vi "Accident Generator.vi"(10 "Accident Number":i32, 11 "Map":i32[][](array[numeric])) -> (2 "Accident Position":T1[](array[typedef]), 3 "Map Out":i32[][](array[numeric]))   [LabVIEW 2015]
uses:
  Data Def/Accident Position.ctl
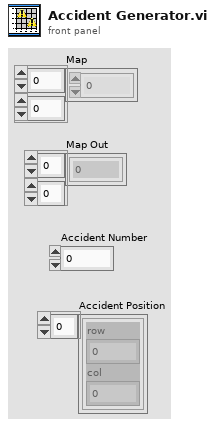
[diagram p1: front panel]
types:
  T1 = typedef "Accident Position.ctl" = cluster{"row":i32, "col":i32}
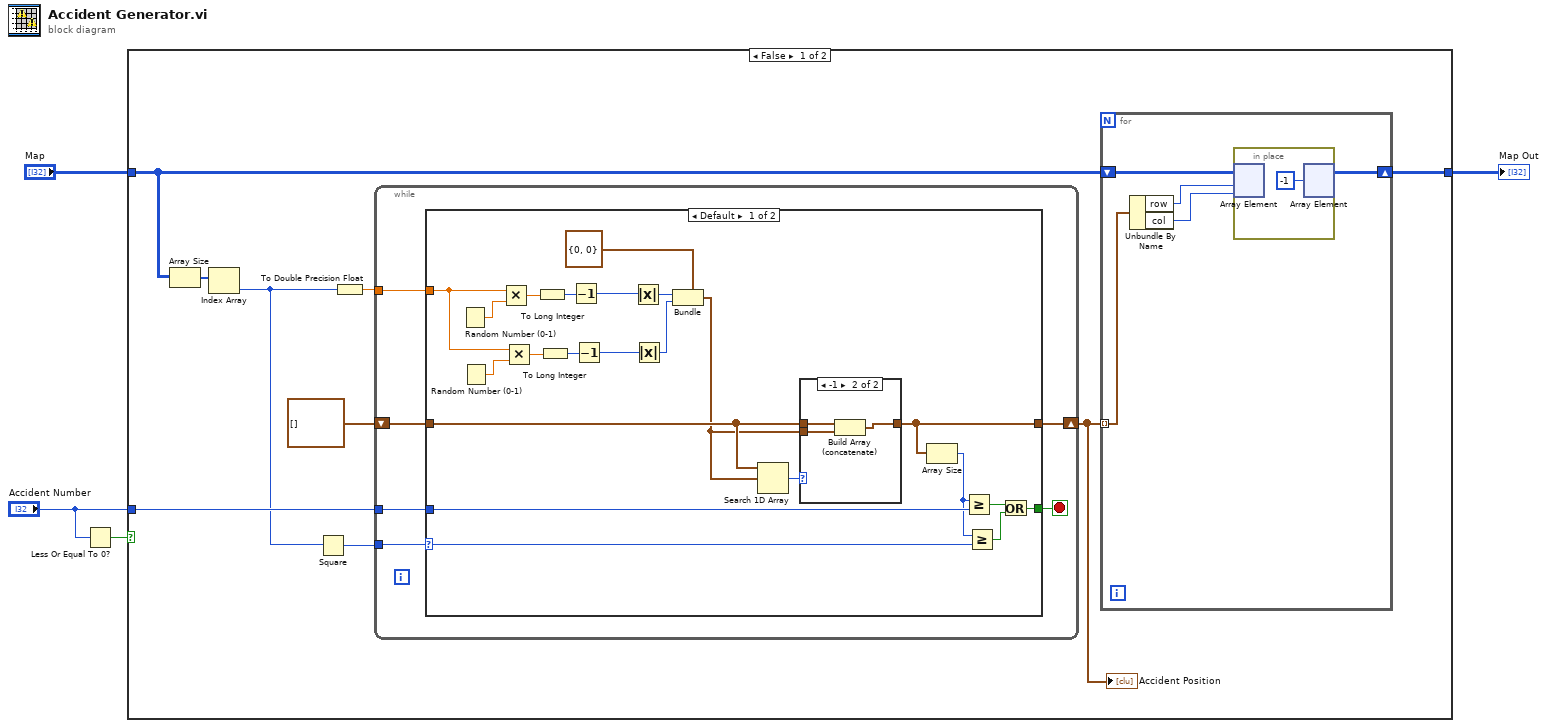
[diagram p0: block diagram]
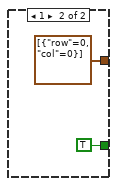
[diagram p3: hidden frame]
diagram:
  n1 = Less Or Equal To 0?(x="Accident Number") -> (x <= 0?=w2:bool)
  n2 = case shown="False" w2 {
    tunnel: "Accident Number" -> [w10 _]
    tunnel: "Map" -> [w6 w54]
    tunnel: [w5 w54] -> w3
    frame False {
      n3 = Array Size(array=w6) -> (size(s)=w13:i32[])
      n4 = Index Array(array=w13) -> (element=w9:i32)  [unwired: 1 in]
      n5 = Square(x=w9) -> (x^2=w8:i32)
      n6 = To Double Precision Float(number=w9) -> (double precision float=w12:dbl)
      n7 = while {
        tunnel: w12 -> [w25]
        shift-right: [w23] -> w7
        shift-left: T1[] [] ("Array") -> [w24]
        tunnel: w10 -> [w22]
        tunnel: w8 -> [w20]
        stop <- w21 stop-if-true
        n8 = case shown="Default" w20 {
          selector: w20 -> [w26 _]
          tunnel: w25 -> [w41 _]
          tunnel: w24 -> [w39 _]
          tunnel: [w36 T1[] [{"row"=0, "col"=0}] ("Array")] -> w23
          tunnel: w22 -> [w31 _]
          tunnel: [w27 TRUE] -> w21
          frame Default {
            n9 = Random Number (0-1)() -> (number: 0 to 1=w47:dbl)
            n10 = Random Number (0-1)() -> (number: 0 to 1=w42:dbl)
            n11 = Multiply(x=w41, y=w47) -> (x*y=w46:dbl)
            n12 = Multiply(x=w41, y=w42) -> (x*y=w43:dbl)
            n13 = To Long Integer(number=w46) -> (32bit integer=w45:i32)
            n14 = To Long Integer(number=w43) -> (32bit integer=w44:i32)
            n15 = Decrement(x=w45) -> (x-1=w35:i32)
            n16 = Decrement(x=w44) -> (x-1=w33:i32)
            n17 = Absolute Value(x=w35) -> (abs(x)=w34:i32)
            n18 = Absolute Value(x=w33) -> (abs(x)=w32:i32)
            n19 = Bundle(cluster=T1 {"row"=0, "col"=0} ("Accident Position"), "row"=w34, "col"=w32) -> (w37:T1)
            n20 = Search 1D Array(1D array=w39, element=w37) -> (index of element=w38:i32)  [unwired: 1 in]
            n21 = case shown="-1" w38 {
              tunnel: w39 -> [w48 w51]
              tunnel: [w48 w49] -> w36
              tunnel: w37 -> [_ w50]
              frame Default {
              }
              frame -1 {
                n22 = Build Array (concatenate)(w51, w50) -> (w49:T1[])
              }
            }
            n23 = Array Size(array=w36) -> (size(s)=w30:i32)
            n24 = Greater Or Equal?(x=w30, y=w31) -> (x >= y?=w29:bool)
            n25 = Greater Or Equal?(x=w30, y=w26) -> (x >= y?=w28:bool)
            n26 = Or(x=w29, y=w28) -> (x .or. y?=w27:bool)
          }
          frame 1 {
          }
        }
      }
      "Accident Position" <- w7
      n27 = for {
        tunnel: w7 -> [w17] mode=indexing
        shift-right: [w14] -> w5
        shift-left: w6 -> [w18]
        n28 = Unbundle By Name(w17) -> ("row"=w16:i32, "col"=w15:i32)
        n29 = in-place {
          n30 = in-place-array #1(w18, w16, w15) -> ()  [unwired: 1 out]
          n31 = in-place-array #1(-1 ("element")) -> (w14:i32[][])  [unwired: 2 out]
        }
      }
    }
    frame True {
    }
  }
  "Map Out" <- w3
